vi "SWTrigEventReference.vi"() -> ()   [LabVIEW 2018]
uses:
  UDP_FGV.ctl
panel:
  in  "SWTRIGEventRef":refnum<event-registration>
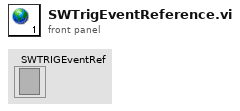
[diagram p1: front panel]
diagram:
